vi "Doppler Moving STFT.vi"() -> ()   [LabVIEW 2022 SP3]
doc: "Performs real-time Joint Time Frequency Analysis (JTFA) using Point By Point STFT. The signal is simulated by a sine wave plus Gaussian noise."
uses:
  <vilib>/measure/mamon.llb/Waveform Peak Detection for N Chan.vi
  <vilib>/measure/NI_MAPro.lvlib
  <vilib>/gmath/NI_Gmath.lvlib
  <vilib>/Analysis/NI_AALBase.lvlib
panel:
  out "BPM":dbl
  out "standard deviation":dbl format="%.4f"
  out "mean":dbl format="%.3f"
  out "Heart rates":dbl[](array[numeric])
  out "Waveform Graph 3":dynamicdata(graph)
  out "Array 4":i32[](array[numeric])
  out "Width 2":i32=4
  in  "time-freq config":cluster{"power of 2":bool, "Nyquist":bool}
  in  "Threshold":dbl=2.0
  in  "Width":i32=4
  in  "stop 2":bool
  out "Number of samples":i32
  out "Extracted":dynamicdata(graph) caption="Signals"
  in  "process data":bool
  in  "time-freq sampling":cluster{"time steps":i32, "freq bins":i32}={"time steps"=64, "freq bins"=128} {"freq bins" format="%0.0f"}
  in  "window info":cluster{"type":u32, "window length":u32}={"type"=2, "window length"=128} {"window length" format="%0.0f"; "type" format="%0.0f"}
  out "Waveform Graph 2":waveform(dbl)(graph)
  out "Locations":cluster{"Locations":dbl[]}[](array[cluster]) {"Locations" format="%.2p"}
  out "Amplitudes":cluster{"Amplitudes":dbl[]}[](array[cluster]) {"Amplitudes" format="%.2p"}
  out "# peaks found":i32[](array[numeric])
  out "Waveform Graph":dbl[](graph)
  out "Array 3":dbl[][](array[numeric])
  out "Array 2":i32[](array[numeric])
  out "Doppler signal":dynamicdata(graph) caption="Signals"
  out "Moving STFT":dbl[][](graph)
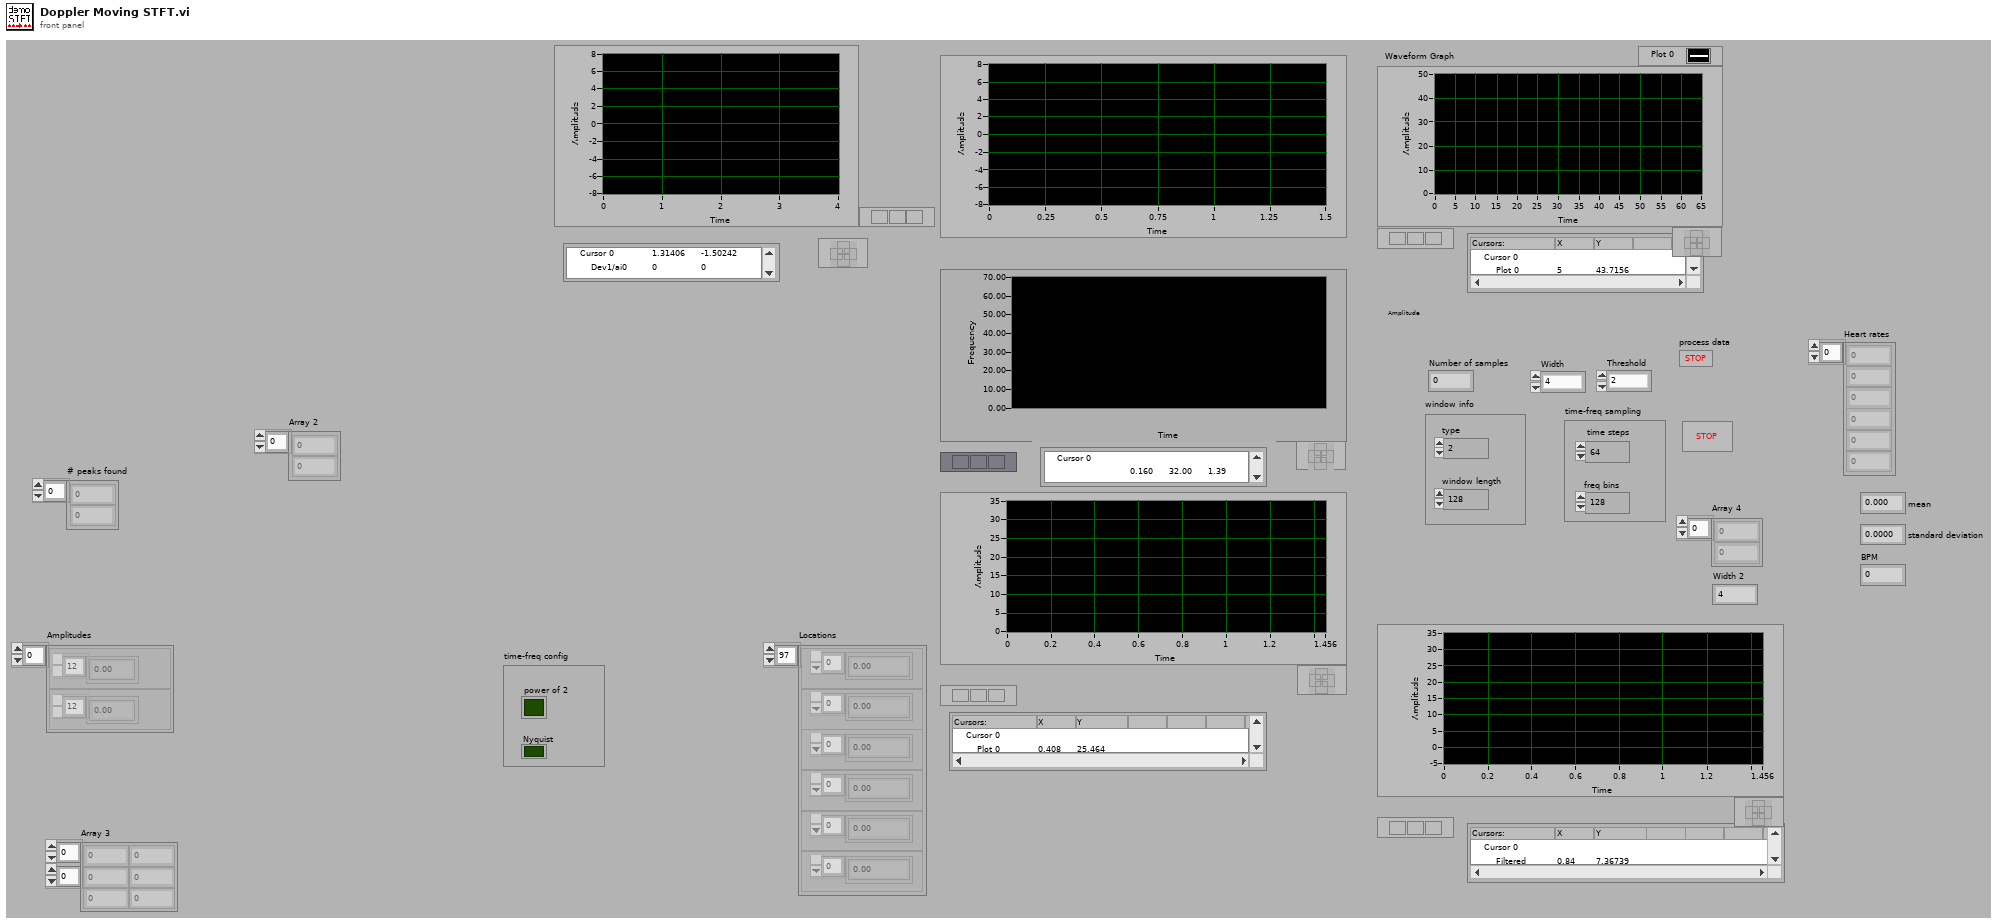
[diagram p1: front panel]
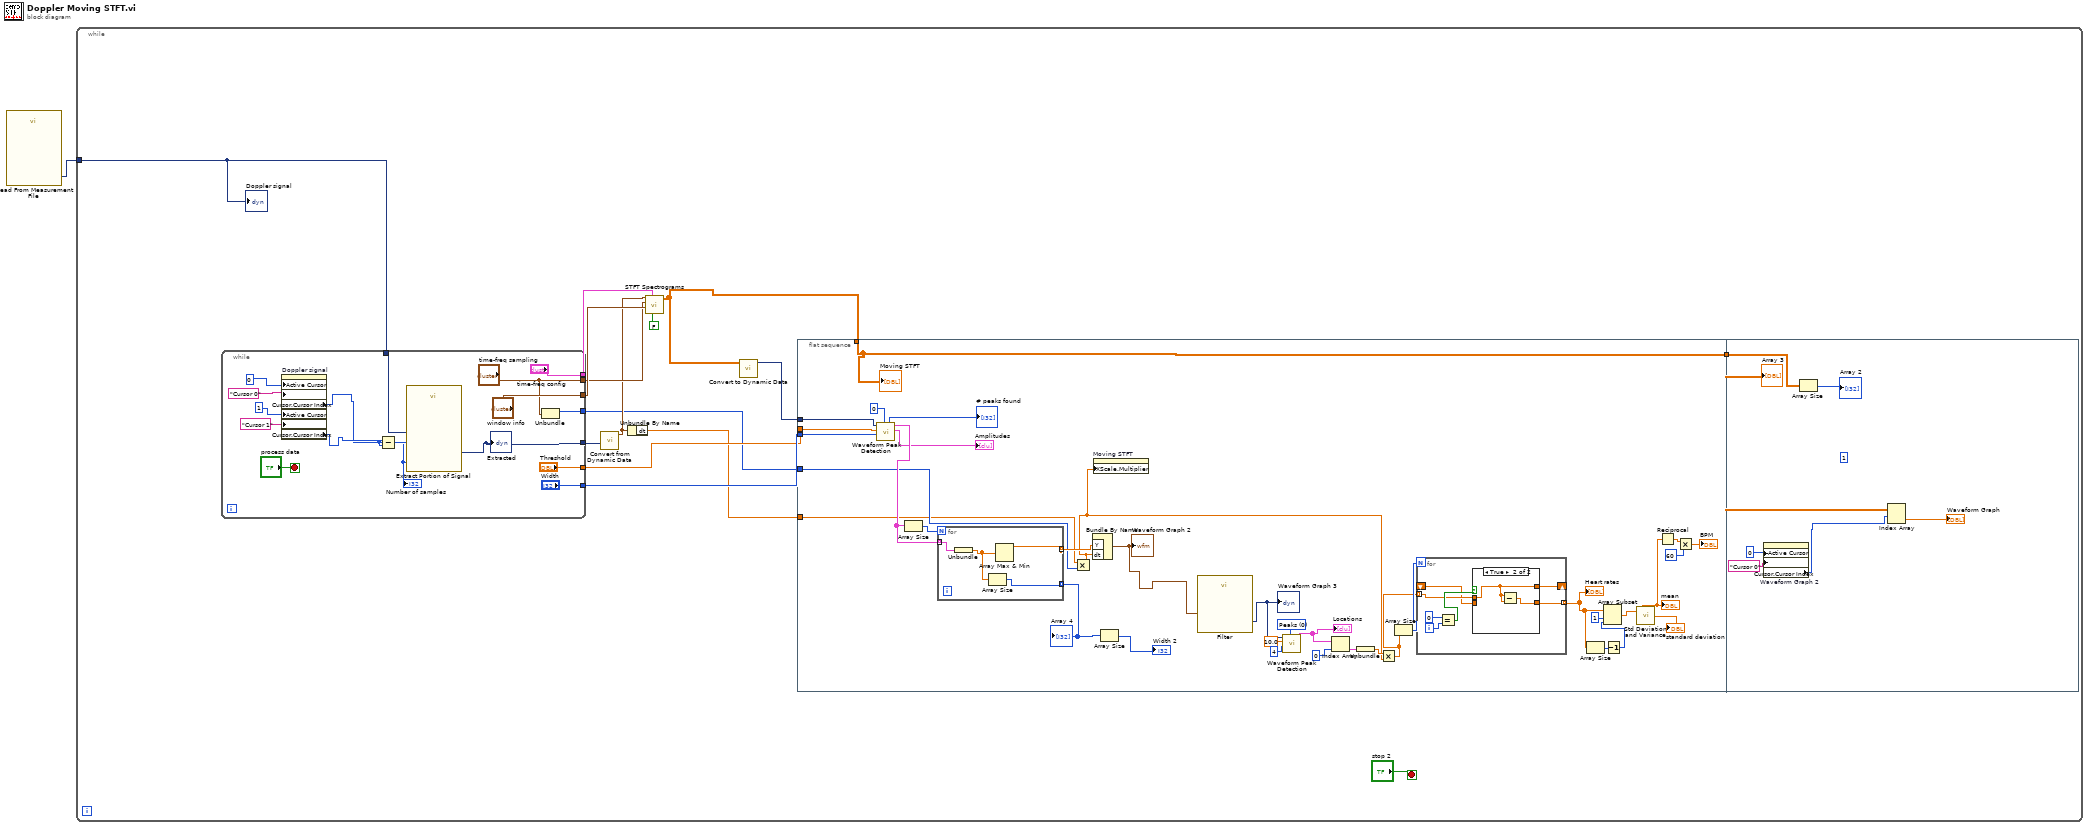
[diagram p0: block diagram]
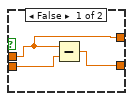
[diagram p2: hidden frame]
diagram:
  n1 = call "Read From Measurement File"() -> ("Signals"=w1:dynamicdata)  [unwired: 4 in, 7 out]
  n2 = while {
    tunnel: w1 -> [w12]
    stop <- "stop 2" stop-if-true
    n3 = while {
      tunnel: w12 -> [w87]
      tunnel: [w79] -> w15
      tunnel: ["window info"] -> w14
      tunnel: ["time-freq sampling"] -> w13
      tunnel: ["Threshold"] -> w6
      tunnel: ["Width"] -> w7
      tunnel: ["time-freq config"] -> w10
      tunnel: [w75] -> w3
      stop <- "process data" stop-if-true
      n4 = property on="Doppler signal" class="WFGraph (strict)"("Active Cursor"=0, "Cursor.Cursor Name"="Cursor 0", "Active Cursor"=1, "Cursor.Cursor Name"="Cursor 1") -> ("Cursor.Cursor Index"=w85:i32, "Cursor.Cursor Index"=w86:i32)  [unwired: 2 in, 2 out]
      n5 = Subtract(x=w86, y=w85) -> (x-y=w84:i32)
      "Number of samples" <- w84
      n6 = call "Extract Portion of Signal"("Samples"=w84, "Begin Sample"=w85, "Signals"=w87) -> ("Section"=w79:dynamicdata)  [unwired: 1 in, 7 out]
      "Extracted" <- w79
      n7 = Unbundle("time-freq sampling") -> ("time steps"=w75:i32)  [unwired: 1 out]
    }
    n8 = call "Convert from Dynamic Data"("Dynamic Data Type"=w15) -> ("Waveform"=w9:waveform(dbl))  [unwired: 1 in, 2 out]
    n9 = Unbundle By Name(w9) -> ("dt"=w2:dbl)
    n10 = call <vilib>:"STFT Spectrograms.vi"("energy conservation?"=FALSE, "time-freq config"=w10, "window info"=w14, "time-freq sampling info"=w13, "X"=w9) -> ("STFT Spectrogram {X}"=w5:dbl[][])  [unwired: 1 in, 5 out]
    n11 = call "Convert to Dynamic Data"("2D Array"=w5) -> ("Dynamic Data Type"=w8:dynamicdata)  [unwired: 3 out]
    n12 = flat-sequence {
      tunnel: w8 -> [w40]
      tunnel: w7 -> [w45]
      tunnel: w6 -> [w44]
      tunnel: w5 -> [w39]
      tunnel: [w39] -> w4
      tunnel: w3 -> [w42]
      tunnel: w2 -> [w41]
      tunnel: w4 -> [w74]
      frame #0 {
        w34 = u16 0 items=["Peaks", "Valleys"] ("peaks/valleys")
        n13 = call-poly <vilib>:"Waveform Peak Detection.vi"("peaks/valleys"=u32 0 ("milliseconds to wait"), "width"=w45, "threshold"=w44, "Signals In"=w40) -> ("Amplitudes"=→"Amplitudes":cluster{"Amplitudes":dbl[]}[], "Locations"=w49:cluster{"Locations":dbl[]}[], "# found"=→"# peaks found":i32[])  [unwired: 3 in, 2 out]
        n14 = Array Size(array=w49) -> (size(s)=w50:i32)
        n15 = for {
          N: w50 -> [_]
          tunnel: w49 -> [w68] mode=indexing
          tunnel: [w67] -> w43 mode=indexing
          tunnel: [w65] -> w51 mode=indexing
          n16 = Unbundle(w68) -> ("Locations"=w66:dbl[])
          n17 = Array Size(array=w66) -> (size(s)=w65:i32)
          n18 = Array Max & Min(array=w66) -> (max value=w67:dbl)  [unwired: 3 out]
        }
        "Array 4" <- w51
        n19 = Multiply(x=w41, y=w42) -> (x*y=w29:dbl)
        n20 = Bundle By Name("Y"=w43, "dt"=w29) -> (w38:waveform(dbl))  [unwired: 1 out]
        "Waveform Graph 2" <- w38
        n21 = property on="Moving STFT" class="IntGraph (strict)"("XScale.Multiplier"=w29) -> ()  [unwired: 2 in, 2 out]
        n22 = Array Size(array=w51) -> (size(s)=→"Width 2":i32)
        n23 = call "Filter"("Signal"=w38) -> ("Filtered Signal"=w37:dynamicdata)  [unwired: 2 in, 8 out]
        "Waveform Graph 3" <- w37
        n24 = call-poly <vilib>:"Waveform Peak Detection.vi"("peaks/valleys"=w34, "width"=4, "threshold"=10.0, "Signals In"=w37) -> ("Locations"=w33:cluster{"Locations":dbl[]}[])  [unwired: 3 in, 4 out]
        "Locations" <- w33
        n25 = Index Array(array=w33, index=0 ("width")) -> (element=w31:cluster{"Locations":dbl[]})
        n26 = Unbundle(w31) -> ("Locations"=w30:dbl[])
        n27 = Multiply(x=w30, y=w29) -> (x*y=w27:dbl[])
        n28 = Array Size(array=w27) -> (size(s)=w28:i32)
        n29 = for {
          N: w28 -> [_]
          tunnel: w27 -> [w56] mode=indexing
          shift-right: [w54] -> _
          shift-left: _ -> [w55]
          tunnel: [w53] -> w24 mode=indexing
          i -> [w59]
          n30 = Equal?(x=0, y=w59) -> (x = y?=w57:bool)
          n31 = case shown="True" w57 {
            tunnel: w56 -> [w61 w64]
            tunnel: [w61 w64] -> w54
            tunnel: w55 -> [w62 _]
            tunnel: [w60 w63] -> w53
            frame False {
              n32 = Subtract(x=w61, y=w62) -> (x-y=w60:dbl)
            }
            frame True {
              n33 = Subtract(x=w64, y=w64) -> (x-y=w63:dbl)
            }
          }
        }
        "Heart rates" <- w24
        n34 = Array Size(array=w24) -> (size(s)=w21:i32)
        n35 = Decrement(x=w21) -> (x-1=w23:i32)
        n36 = Array Subset(array=w24, index=1, length=w23) -> (w25:dbl[])
        n37 = call <vilib>:"Std Deviation and Variance.vi"("X"=w25) -> ("mean"=w20:dbl, "standard deviation"=→"standard deviation":dbl)  [unwired: 1 in, 1 out]
        "mean" <- w20
        n38 = Reciprocal(x=w20) -> (1/x=w19:dbl)
        n39 = Multiply(x=w19, y=60 ("index")) -> (x*y=→"BPM":dbl)
        "Moving STFT" <- w39
      }
      frame #1 {
        (unwired) u32 1 ("milliseconds to wait")
        n40 = property on="Waveform Graph 2" class="WFGraph (strict)"("Active Cursor"=0, "Cursor.Cursor Name"="Cursor 0") -> ("Cursor.Cursor Index"=w69:i32)  [unwired: 2 in, 2 out]
        n41 = Array Size(array=w74) -> (size(s)=→"Array 2":i32[])
        n42 = Index Array(array=w74, index (row)=w69) -> (element=→"Waveform Graph":dbl[])  [unwired: 1 in]
        "Array 3" <- w74
      }
    }
    "Doppler signal" <- w12
  }
